vi "New wavelength array.vi"(7 "Monochromator in":T1={"Type"=enum."Oriel", "Wavelength (nm)"=0.0, "Grating, gr/mm"=enum."2400", "Grating mode"=enum."IR", "Spectrum mode"={"Spectrum mode?"=FALSE, "Start wavelength (nm)"=0.0, "End wavelength (nm)"=0.0, "Wavelength step (nm)"=0.0, "Wavelength array"=[], "array index"=0}, "PTI"={"Delay before read (ms)"=0, "Mono 1"={"Timeout (ms)"=0, "Resource Name"="", "Baud Rate"=0, "Data Bits"=0, "Parity"=0, "Stop Bits"=0, "Flow Control"=0}, "Mono 2"={"Timeout (ms)"=0, "Resource Name"="", "Baud Rate"=0, "Data Bits"=0, "Parity"=0, "Stop Bits"=0, "Flow Control"=0}, "Two PTI Monochromators?"=FALSE}, "Oriel (custom)"={"reference"=refnum}, "Force wavelength confirmation (PTI)?"=FALSE} {"PTI"."Mono 2"."Flow Control" items=["1.0"=10, "1.5"=15, "2.0"=20]; "PTI"."Mono 2"."Stop Bits" items=["None", "Odd", "Even", "Mark", "Space"]; "PTI"."Mono 2"."Parity" items=["None", "Odd", "Even", "Mark", "Space"]; "PTI"."Mono 1"."Flow Control" items=["1.0"=10, "1.5"=15, "2.0"=20]; "PTI"."Mono 1"."Stop Bits" items=["None", "Odd", "Even", "Mark", "Space"]; "PTI"."Mono 1"."Parity" items=["None", "Odd", "Even", "Mark", "Space"]}, 8 "Error In":errorcluster) -> (0 "Error Out":errorcluster, 5 "Monochromator out":T1={"Type"=enum."Oriel", "Wavelength (nm)"=0.0, "Grating, gr/mm"=enum."2400", "Grating mode"=enum."IR", "Spectrum mode"={"Spectrum mode?"=FALSE, "Start wavelength (nm)"=0.0, "End wavelength (nm)"=0.0, "Wavelength step (nm)"=0.0, "Wavelength array"=[], "array index"=0}, "PTI"={"Delay before read (ms)"=0, "Mono 1"={"Timeout (ms)"=0, "Resource Name"="", "Baud Rate"=0, "Data Bits"=0, "Parity"=0, "Stop Bits"=0, "Flow Control"=0}, "Mono 2"={"Timeout (ms)"=0, "Resource Name"="", "Baud Rate"=0, "Data Bits"=0, "Parity"=0, "Stop Bits"=0, "Flow Control"=0}, "Two PTI Monochromators?"=FALSE}, "Oriel (custom)"={"reference"=refnum}, "Force wavelength confirmation (PTI)?"=FALSE} {"PTI"."Mono 2"."Flow Control" items=["1.0"=10, "1.5"=15, "2.0"=20]; "PTI"."Mono 2"."Stop Bits" items=["None", "Odd", "Even", "Mark", "Space"]; "PTI"."Mono 2"."Parity" items=["None", "Odd", "Even", "Mark", "Space"]; "PTI"."Mono 1"."Flow Control" items=["1.0"=10, "1.5"=15, "2.0"=20]; "PTI"."Mono 1"."Stop Bits" items=["None", "Odd", "Even", "Mark", "Space"]; "PTI"."Mono 1"."Parity" items=["None", "Odd", "Even", "Mark", "Space"]})   [LabVIEW 2017, in "Monochromator.lvlib"]
uses:
  Monochromator.lvlib
  Controls/Params.ctl
  Controls/Type.ctl
  Controls/GratingValues.ctl
  Controls/Grating.ctl
  PTI/Controls/Params.ctl
  Controls/VISA parameters.ctl
  Custom Oriel drivers/Controls/Params.ctl
  C:/Project Work/icl-optical-software-rewrite/Optical Software Code Simplified/Modules/Monochromator/Cornerstone.dll
  Cornerstone.dll
  Controls/Errors.ctl
  <vilib>/Utility/error.llb/Error Cluster From Error Code.vi
  <vilib>/ErrorRing/Error Ring.xnode
  Serial comms/Serial comms.lvlib
  PTI/PTI.lvlib
  Custom Oriel drivers/Oriel (custom drivers).lvlib
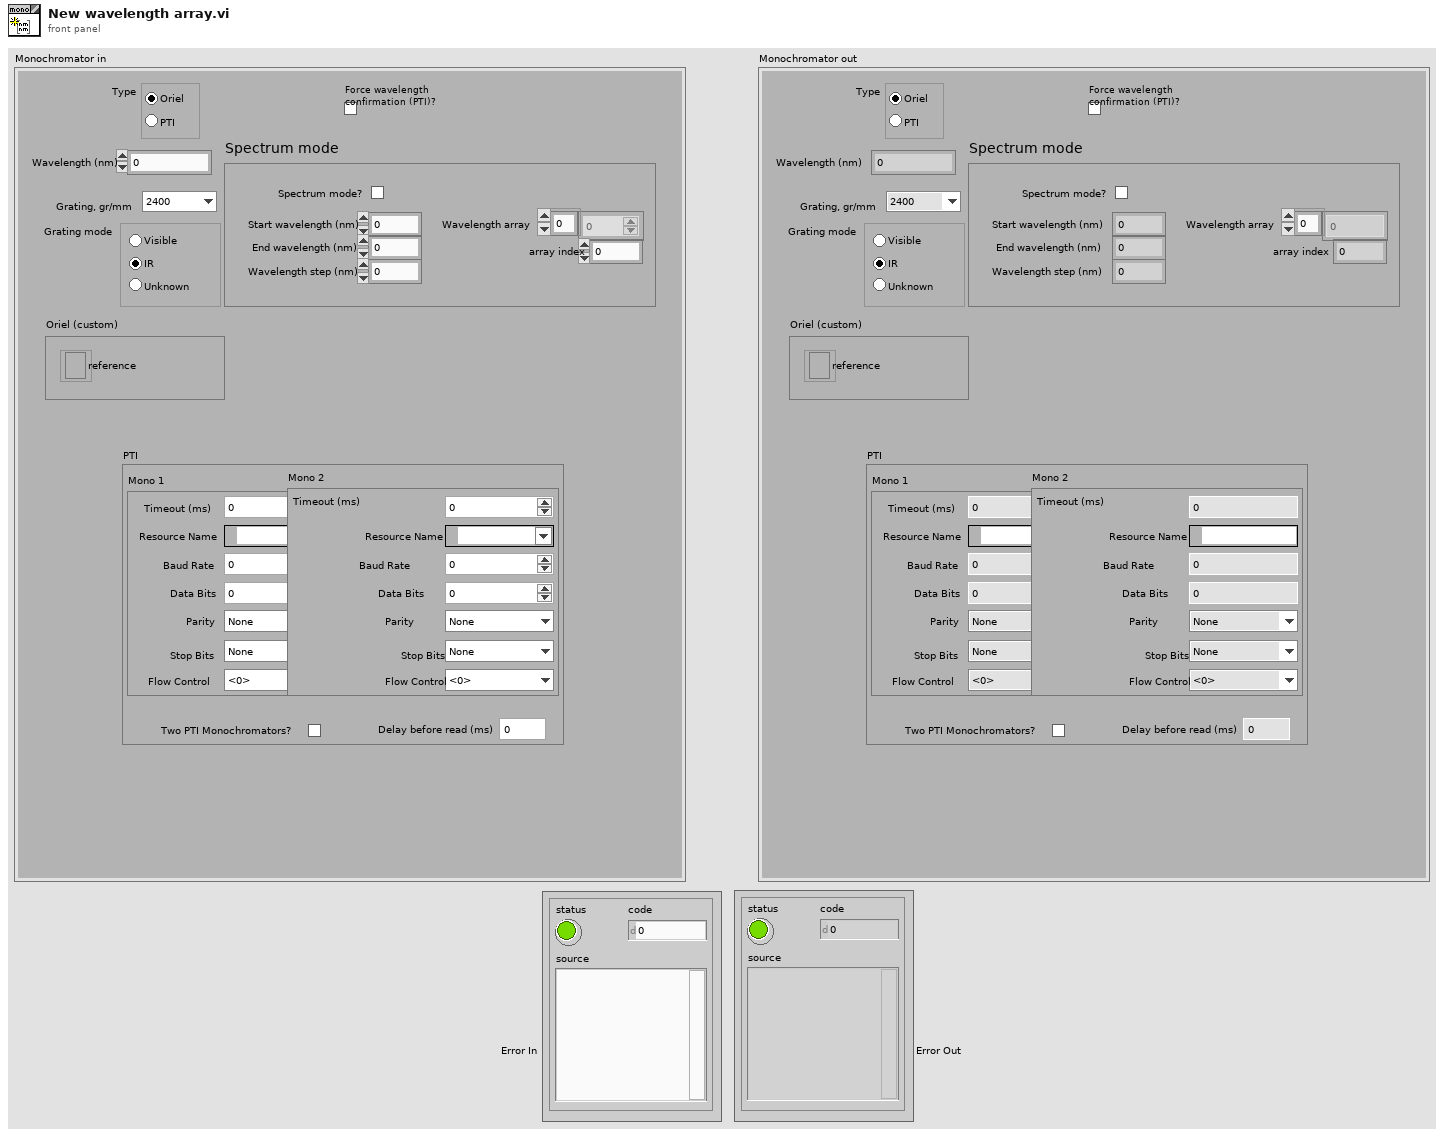
[diagram p1: front panel]
types:
  T1 = typedef "Monochromator.lvlib/Params.ctl" = cluster{"Type":T2, "Wavelength (nm)":dbl, "Grating, gr/mm":T3, "Grating mode":T4, "Spectrum mode":cluster{"Spectrum mode?":bool, "Start wavelength (nm)":dbl, "End wavelength (nm)":dbl, "Wavelength step (nm)":dbl, "Wavelength array":dbl[], "array index":u32}, "PTI":T5, "Oriel (custom)":T7, "Force wavelength confirmation (PTI)?":bool}
  T2 = typedef "Monochromator.lvlib/Type.ctl" = enum32{"Oriel", "PTI"}
  T3 = typedef "Monochromator.lvlib/GratingValues.ctl" = enum16{"2400", "1800", "1200", "600", "300", "150"}
  T4 = typedef "Monochromator.lvlib/Grating.ctl" = enum32{"Unknown", "Visible", "IR"}
  T5 = typedef "Monochromator.lvlib/PTI.lvlib/Params.ctl" = cluster{"Delay before read (ms)":u32, "Mono 1":T6, "Mono 2":T6, "Two PTI Monochromators?":bool}
  T6 = typedef "Serial comms.lvlib/VISA parameters.ctl" = cluster{"Timeout (ms)":u32, "Resource Name":refnum<visa-resource-name>, "Baud Rate":u32, "Data Bits":u16, "Parity":u16, "Stop Bits":u16, "Flow Control":u16}
  T7 = typedef "Monochromator.lvlib/Oriel (custom drivers).lvlib/Params.ctl" = cluster{"reference":refnum<k24>}
  T8 = cluster{"Spectrum mode?":bool, "Start wavelength (nm)":dbl, "End wavelength (nm)":dbl, "Wavelength step (nm)":dbl, "Wavelength array":dbl[], "array index":u32}
  T9 = typedef "Monochromator.lvlib/Errors.ctl" = cluster{"Invalid wavelength":errorcluster, "Empty wavelength array":errorcluster, "Index out of range":errorcluster}
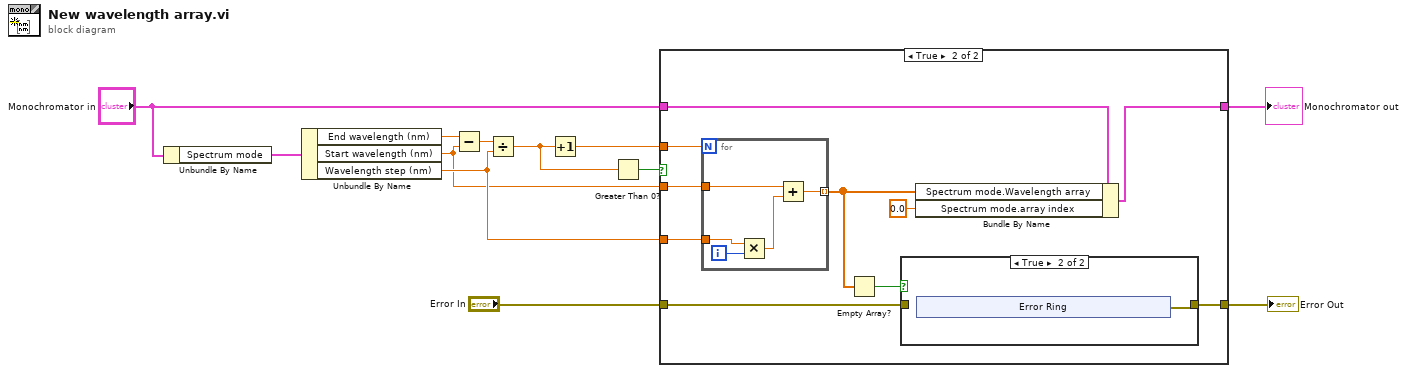
[diagram p0: block diagram]
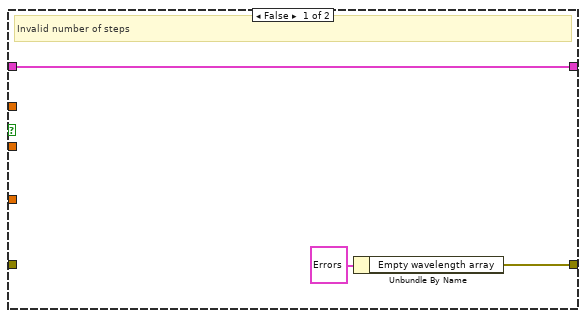
[diagram p2: hidden frame]
diagram:
  n1 = Unbundle By Name("Monochromator in") -> ("Spectrum mode"=w3:T8)
  n2 = Unbundle By Name(w3) -> ("End wavelength (nm)"=w9:dbl, "Start wavelength (nm)"=w11:dbl, "Wavelength step (nm)"=w12:dbl)
  n3 = Subtract(x=w9, y=w11) -> (x-y=w10:dbl)
  n4 = Divide(x=w10, y=w12) -> (x/y=w5:dbl)
  n5 = Increment(x=w5) -> (x+1=w4:dbl)
  n6 = Greater Than 0?(x=w5) -> (x > 0?=w6:bool)
  n7 = case shown="True" w6 {
    tunnel: "Monochromator in" -> [w15 w18]
    tunnel: [w15 w17] -> w1
    tunnel: w12 -> [_ w25]
    tunnel: w11 -> [_ w24]
    tunnel: w4 -> [_ w23]
    tunnel: [w14 w20] -> w8
    tunnel: "Error In" -> [_ w19]
    frame False {
      # "Invalid number of steps"
      n8 = Unbundle By Name(T9 {"Invalid wavelength"={"status"=FALSE, "code"=5100, "source"="An invalid wavelength was received in the Monochromator module."}, "Empty wavelength array"={"status"=FALSE, "code"=5101, "source"="Invalid start/step/end wavelengths—an empty array was generated."}, "Index out of range"={"status"=FALSE, "code"=5101, "source"="Invalid start/step/end wavelengths"}} ("Monochromator errors")) -> ("Empty wavelength array"=w14:errorcluster)
    }
    frame True {
      n9 = for {
        N: w23 -> [_]
        tunnel: w24 -> [w37]
        tunnel: w25 -> [w35]
        tunnel: [w33] -> w22 mode=indexing
        i -> [w36]
        n10 = Multiply(x=w35, y=w36) -> (x*y=w34:dbl)
        n11 = Add(x=w37, y=w34) -> (x+y=w33:dbl)
      }
      n12 = Empty Array?(array=w22) -> (empty?=w21:bool)
      n13 = case shown="True" w21 {
        tunnel: [w26 w27] -> w20
        tunnel: w19 -> [w26 _]
        frame False {
        }
        frame True {
          n14 = xnode "Error Ring"() -> ("error out"=w27:errorcluster)
        }
      }
      n15 = Bundle By Name(cluster=w18, "Spectrum mode.Wavelength array"=w22, "Spectrum mode.array index"=0.0) -> (w17:T1)
    }
  }
  "Monochromator out" <- w1
  "Error Out" <- w8
